vi "Get Top Entities.vi"() -> ()   [LabVIEW 2014]
uses:
  types/Entities.ctl
  <vilib>/Utility/traverseref.llb/VI Scripting - Traverse.lvlib
  <vilib>/Utility/traverseref.llb/TRef TravTarget.ctl
panel:
  out "# of Numeric":i32
  out "# of Tunnels":i32
  out "References":refnum<vi>[](array[refnum])
  out "Data Type":string[][](array[string])
  out "Array 2":variant[](array[variant])
  out "Array":string[](array[string])
  out "Connector Pane Terminals Names":string[](array[string])
  out "size(s)":i32
  out "__return":string
  in  "__args":cluster{"targetVi":string}={"targetVi"="c:\\Users\\lubo\\Documents\\LabView\\LabVIEW-Universal-Transcriptor\\Test\\Example Test 1.vi"}
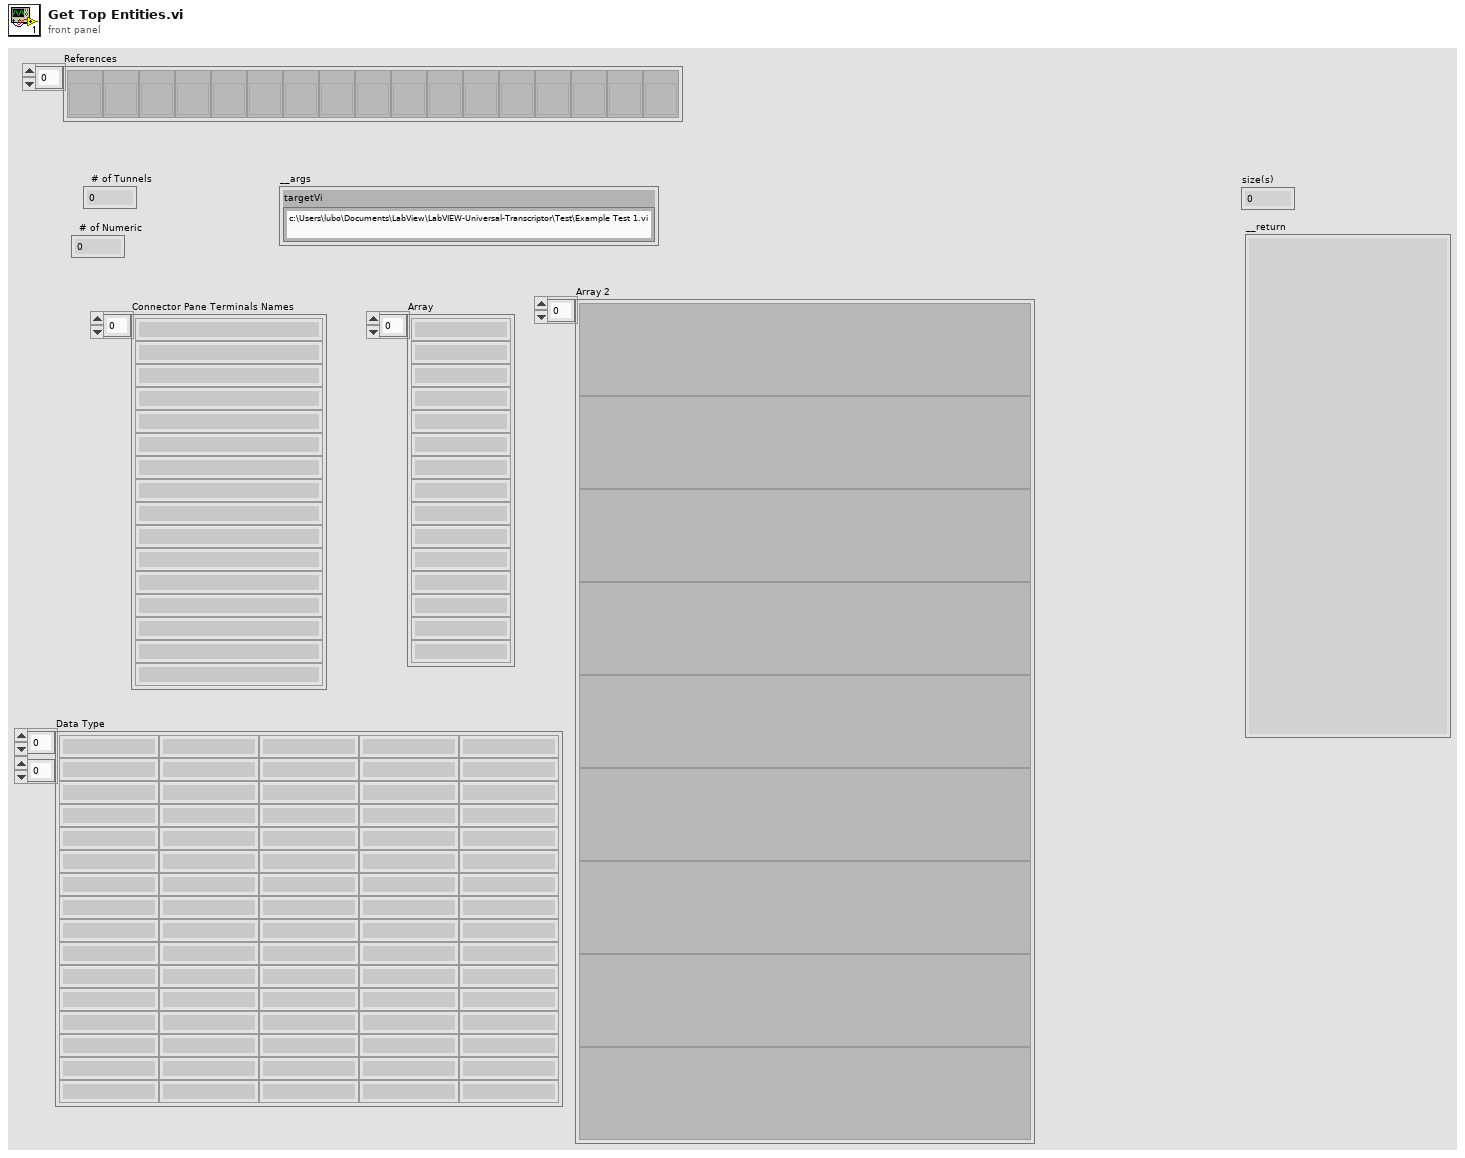
[diagram p1: front panel]
types:
  T1 = typedef "Entities.ctl" = string
  T2 = typedef "TRef TravTarget.ctl" = enum16{"FP", "BD", "Other"}
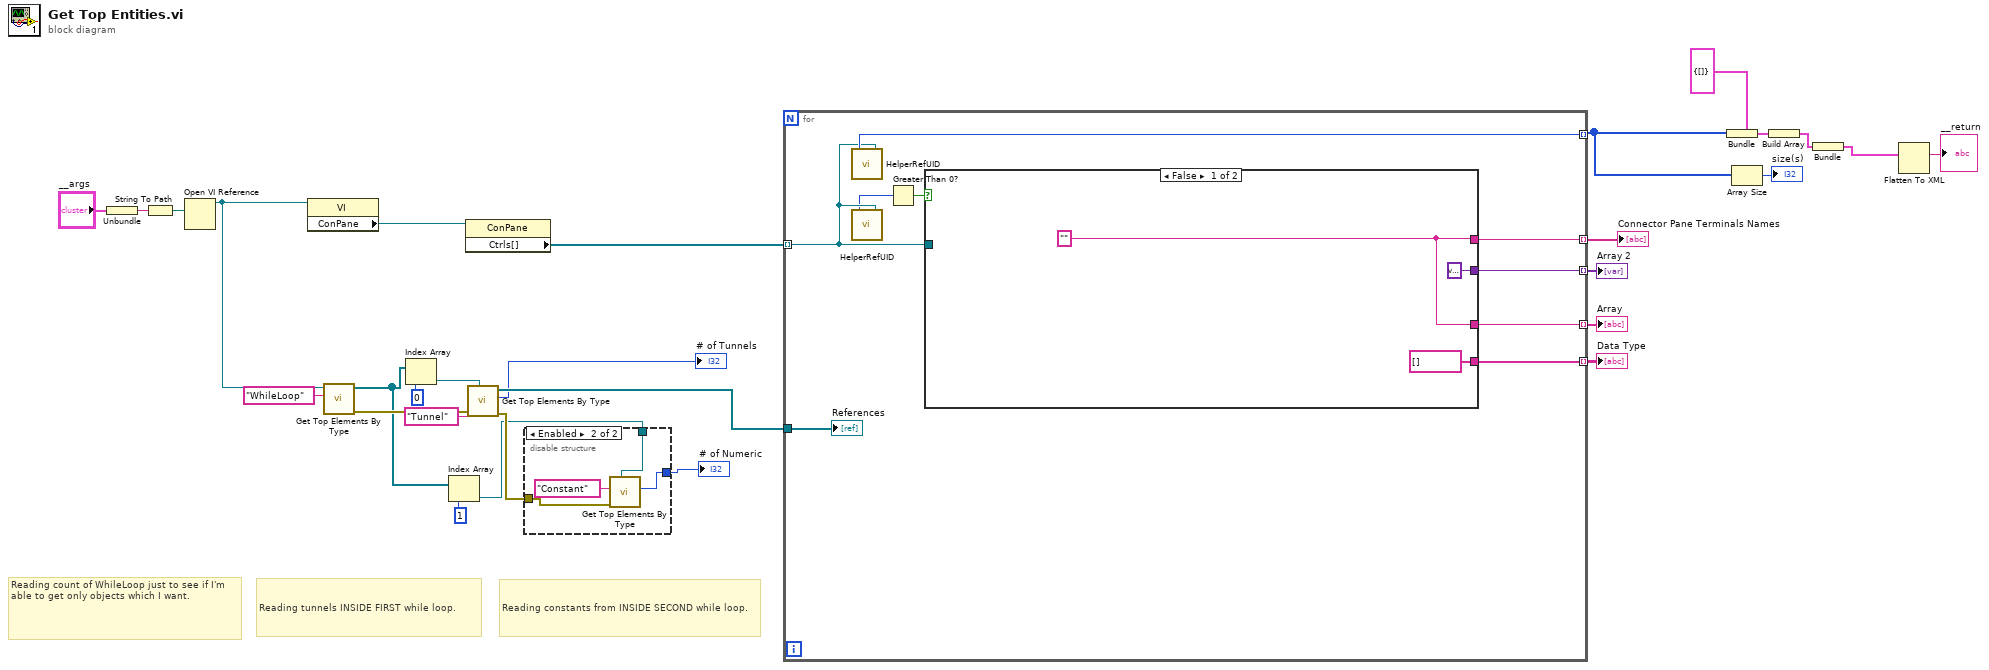
[diagram p0: block diagram]
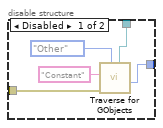
[diagram p2: hidden frame]
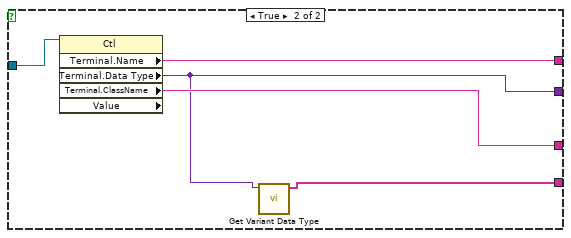
[diagram p3: hidden frame]
diagram:
  # "Reading constants from INSIDE SECOND while loop."
  # "Reading tunnels INSIDE FIRST while loop."
  # "Reading count of WhileLoop just to see if I'm\nable to get only objects which I want."
  n1 = Unbundle("__args") -> ("targetVi"=w28:string)
  n2 = String To Path(string=w28) -> (path=w26:path)
  n3 = Open VI Reference(vi path=w26) -> (vi reference=w13:refnum<vi>)  [unwired: 5 in, 1 out]
  n4 = property class="VI"(reference=w13) -> ("ConPane"=w18:refnum<vi>)  [unwired: 1 in, 2 out]
  n5 = call "Get Top Elements By Type.vi"("type"=T1 "WhileLoop", "VI in"=w13) -> ("error out"=w11:errorcluster, "References"=w4:refnum<vi>[])  [unwired: 7 in, 1 out]
  n6 = Index Array(array=w4, index=0) -> (element=w7:refnum<vi>)
  n7 = Index Array(array=w4, index=1) -> (element=w3:refnum<vi>)
  n8 = property class="ConPane"(reference=w18) -> ("Ctrls[]"=w25:refnum<vi>[])  [unwired: 1 in, 2 out]
  n9 = call "Get Top Elements By Type.vi"("Other Refnum"=w7, "error in (no error)"=w11, "type"=T1 "Tunnel") -> ("error out"=w8:errorcluster, "# of Refs"=→"# of Tunnels":i32, "References"=w10:refnum<vi>[])  [unwired: 6 in]
  n10 = disable-structure shown="Enabled" {
    disable-tunnel: w8 -> [w33 w38]
    disable-tunnel: [w32 w36] -> w6
    disable-tunnel: w3 -> [w30 w37]
    frame Disabled {
      n11 = call <vilib>:"Traverse for GObjects.vi"("Other Refnum"=w30, "Traverse Target"=TRef_TravTarget."Other", "error in (no error)"=w33, "Class Name"="Constant") -> ("# of Refs"=w32:i32)  [unwired: 4 in, 3 out]
    }
    frame Enabled {
      n12 = call "Get Top Elements By Type.vi"("Other Refnum"=w37, "error in (no error)"=w38, "type"=T1 "Constant") -> ("# of Refs"=w36:i32)  [unwired: 6 in, 2 out]
    }
  }
  "# of Numeric" <- w6
  n13 = for {
    tunnel: w25 -> [w45] mode=indexing
    tunnel: [w47] -> w20 mode=indexing
    tunnel: [w46] -> w17 mode=indexing
    tunnel: [w42] -> w15 mode=indexing
    tunnel: [w41] -> w16 mode=indexing
    tunnel: [w40] -> w14 mode=indexing
    tunnel: w10 -> [w39]
    n14 = call "HelperRefUID.vi"("Text in"=w45) -> ("UID"=w47:i32)
    n15 = call "HelperRefUID.vi"("Text in"=w45) -> ("UID"=w44:i32)
    n16 = Greater Than 0?(x=w44) -> (x > 0?=w43:bool)
    n17 = case shown="False" w43 {
      tunnel: [w50 w55] -> w46
      tunnel: w45 -> [_ w54]
      tunnel: [variant ("Terminal.Data Type") w52] -> w42
      tunnel: [w50 w53] -> w41
      tunnel: [string[] [] ("Data Type") w51] -> w40
      frame False {
        w50 = "" ("Desc")
      }
      frame True {
        n18 = property class="Ctl" props=["Terminal", "Name", "Terminal", "Data Type", "Terminal", "ClassName", "Value"](reference=w54) -> ("Terminal.Name"=w55:string, "Terminal.Data Type"=w52:variant, "Terminal.ClassName"=w53:string)  [unwired: 1 in, 3 out]
        n19 = call "Get Variant Data Type.vi"("variant"=w52) -> ("Data Type"=w51:string[])  [unwired: 10 in]
      }
    }
    "References" <- w39
  }
  "Connector Pane Terminals Names" <- w17
  "Array" <- w16
  "Array 2" <- w15
  "Data Type" <- w14
  n20 = Bundle(cluster=cluster{"Controls[]":i32[]} {"Controls[]"=[]} ("ConnectorPane"), "Controls[]"=w20) -> (w22:cluster{"Controls[]":i32[]})
  n21 = Array Size(array=w20) -> (size(s)=→"size(s)":i32)
  n22 = Build Array(w22) -> (w21:cluster{"Controls[]":i32[]}[])
  n23 = Bundle(w21) -> (w24:cluster{cluster{"Controls[]":i32[]}[]})  [unwired: 1 in]
  n24 = Flatten To XML(anything=w24) -> (xml string=→"__return":string)
